vi "Read Module Settings.vi"(0 "class data in":refnum<class "MB_MODULE.lvclass">, 11 "error in (no error)":errorcluster) -> (4 "class data out":refnum<class "MB_MODULE.lvclass">, 15 "error out":errorcluster)   [LabVIEW 2019, in "MB_MODULE.lvclass"]
uses:
  MB_MODULE.lvclass
  Module Settings.ctl
panel:
  out "Settings":T1
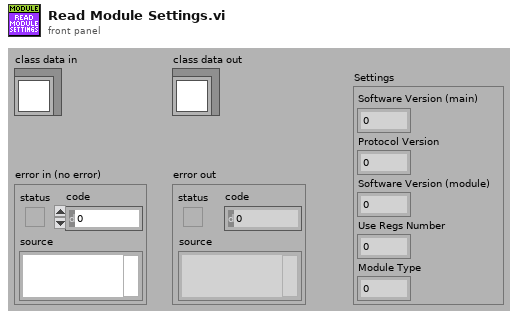
[diagram p1: front panel]
types:
  T1 = typedef "MB_MODULE.lvclass/Module Settings.ctl" = cluster{"Software Version (main)":u16, "Protocol Version":u16, "Software Version (module)":u16, "Use Regs Number":u16, "Module Type":u16}
  T2 = cluster{"register values[0]":u16, "register values[1]":u16, "register values[2]":u16, "register values[3]":u16, "register values[4]":u16}
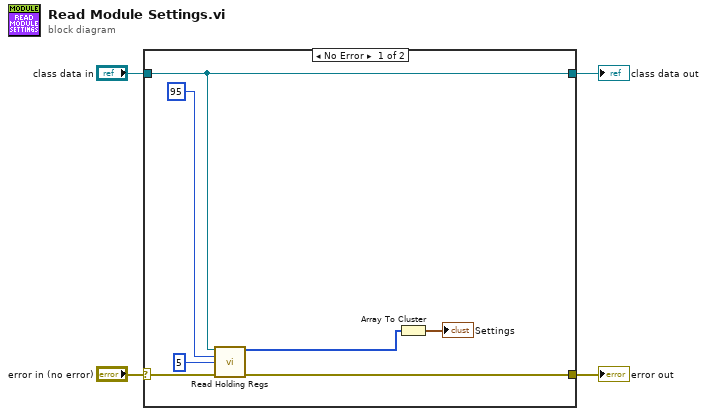
[diagram p0: block diagram]
diagram:
  n1 = case shown="No Error" "error in (no error)" {
    selector: "error in (no error)" -> [w8 w13]
    tunnel: [w7 w13] -> w3
    tunnel: "class data in" -> [w11 w12]
    tunnel: [w11 w12] -> w1
    frame No Error {
      n2 = call-dynamic "Read Holding Regs.vi"("reference in"=w11, "starting address"=u16 95, "number of inputs"=u16 5, "error in (no error)"=w8) -> ("register values"=w6:u16[], "error out"=w7:errorcluster)  [unwired: 10 in]
      n3 = Array To Cluster(array=w6) -> (cluster=→"Settings":T2)
    }
    frame Error {
    }
  }
  "error out" <- w3
  "class data out" <- w1
